vi "URLDecode.vi"(2 "URL":string) -> (7 "Decoded":string)   [LabVIEW 2023]
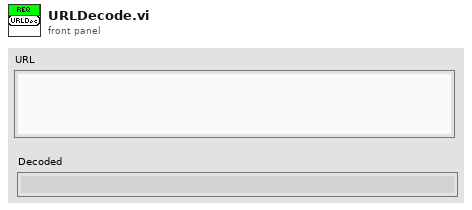
[diagram p1: front panel]
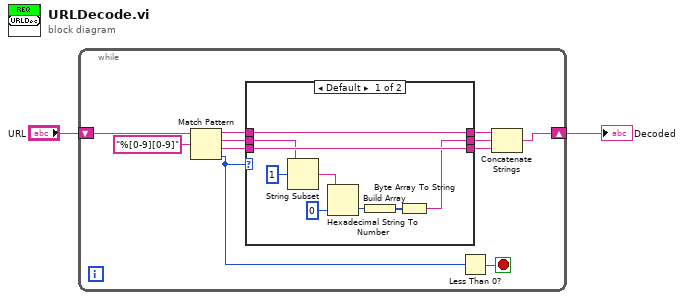
[diagram p0: block diagram]
diagram:
  n1 = while {
    shift-right: [w5] -> w1
    shift-left: "URL" -> [w12]
    stop <- w4 stop-if-true
    n2 = Match Pattern(string=w12, regular expression="%[0-9][0-9]") -> (before substring=w11:string, match substring=w10:string, after substring=w9:string, offset past match=w3:i32)  [unwired: 1 in]
    n3 = case shown="Default" w3 {
      tunnel: w11 -> [w22 w25]
      tunnel: w10 -> [w20 w24]
      tunnel: w9 -> [w21 w23]
      tunnel: [w22 w25] -> w8
      tunnel: [w15 w24] -> w7
      tunnel: [w21 w23] -> w6
      frame Default {
        n4 = String Subset(string=w20, offset (0)=1) -> (substring=w14:string)  [unwired: 1 in]
        n5 = Hexadecimal String To Number(string=w14, default (0uL)=u8 0 ("default value 1")) -> (number=w17:u8)  [unwired: 1 in, 1 out]
        n6 = Build Array(w17) -> (w16:u8[])
        n7 = Byte Array To String(unsigned byte array=w16) -> (string=w15:string)
      }
      frame -1 {
      }
    }
    n8 = Less Than 0?(x=w3) -> (x < 0?=w4:bool)
    n9 = Concatenate Strings(w8, w7, w6) -> (w5:string)
  }
  "Decoded" <- w1
